vi "Configure Marker Frequency.vi"(8 "error in (no error)":errorcluster, 9 "Marker Frequency":dbl, 10 "Marker Number":u8=1, 11 "VNA-FieldFox in":refnum<class "VNA-FieldFox.lvclass">) -> (0 "error out":errorcluster, 3 "VNA-FieldFox out":refnum<class "VNA-FieldFox.lvclass">)   [LabVIEW 2020, in "VNA-FieldFox.lvclass"]
doc: "Configure the marker frequency.\nThe marker is always set on the current active trace."
uses:
  VNA-FieldFox.lvclass
  Vector Network Analyzer.lvclass
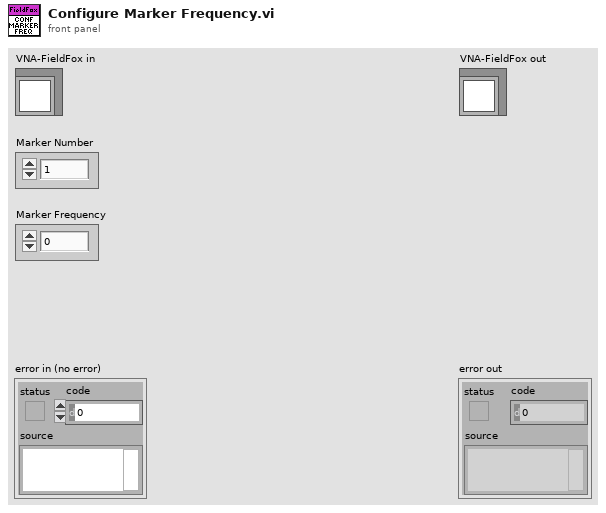
[diagram p1: front panel]
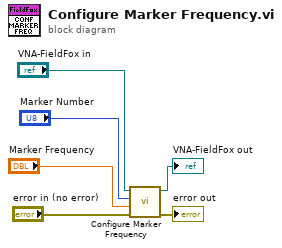
[diagram p0: block diagram]
diagram:
  n1 = call-parent "Configure Marker Frequency.vi"("error in (no error)"="error in (no error)", "Marker Frequency"="Marker Frequency", "Marker Number"="Marker Number", "Vector Network Analyzer in"="VNA-FieldFox in") -> ("error out"=→"error out":errorcluster, "Vector Network Analyzer out"=→"VNA-FieldFox out":refnum<class "VNA-FieldFox.lvclass">)  [unwired: 6 in]
